vi "Create Server.vi"(5 "Server Key File (.key)":path, 7 "Server Certificate File (.crt)":path, 8 "error in (no error)":errorcluster, 11 "Server Address":string) -> (0 "error out":errorcluster, 3 "gRPC Server out":refnum<class "HVC4.lvclass">)   [LabVIEW 2019, in "HVC4.lvlib" / "HVC4.lvclass"]
uses:
  HVC4.lvclass
  HVC4.lvclass/HVC4.ctl
  gRPC lvSupport/gprc-lvsupport.lvlib
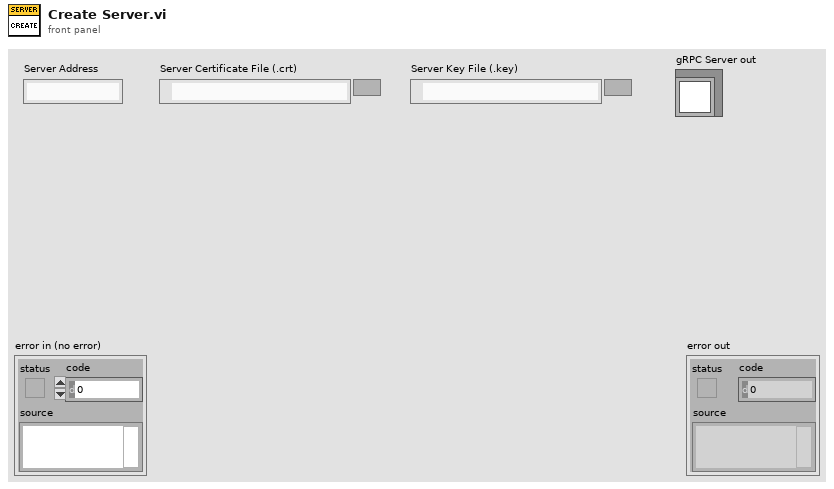
[diagram p1: front panel]
types:
  T1 = typedef "HVC4.lvlib/gprc-lvsupport.lvlib/grpcId.ctl" = u64
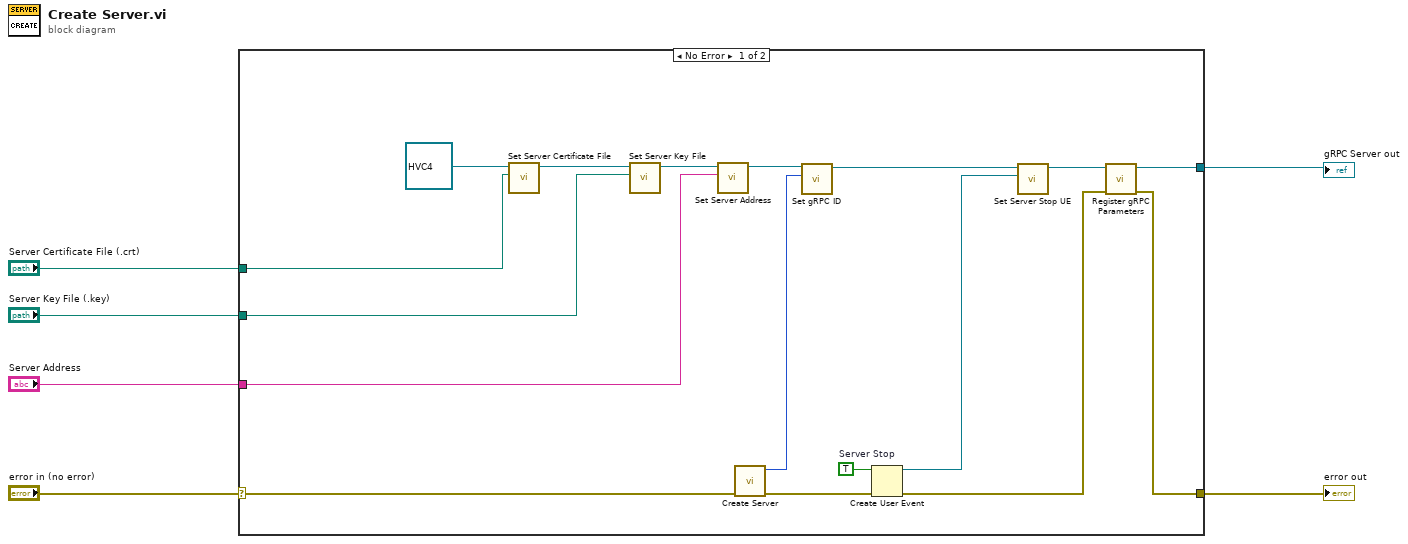
[diagram p0: block diagram]
diagram:
  n1 = case shown="No Error" "error in (no error)" {
    selector: "error in (no error)" -> [w23 w24]
    tunnel: [w7 w24] -> w5
    tunnel: [w9 _] -> w4
    tunnel: "Server Certificate File (.crt)" -> [w18 _]
    tunnel: "Server Key File (.key)" -> [w17 _]
    tunnel: "Server Address" -> [w16 _]
    frame No Error {
      w14 = TRUE  # Server Stop
      n2 = call "Set Server Certificate File.vi"("Server Certificate File (.crt)"=w18, "OOP Server in"=refnum<class "HVC4.lvclass"> refnum ("OOP Server out")) -> ("OOP Server out"=w21:refnum<class "HVC4.lvclass">)  [unwired: 9 in]
      n3 = call "Set Server Key File.vi"("Server Key File (.key)"=w17, "OOP Server in"=w21) -> ("OOP Server out"=w20:refnum<class "HVC4.lvclass">)  [unwired: 9 in]
      n4 = call "Set Server Address.vi"("Server Address"=w16, "OOP Server in"=w20) -> ("OOP Server out"=w19:refnum<class "HVC4.lvclass">)  [unwired: 9 in]
      n5 = call "Create Server.vi"("error in (no error)"=w23) -> ("error out"=w12:errorcluster, "gRPCid"=w15:T1)  [unwired: 9 in]
      n6 = call "Set gRPC ID.vi"("gRPC ID"=w15, "OOP Server in"=w19) -> ("OOP Server out"=w13:refnum<class "HVC4.lvclass">)  [unwired: 9 in]
      n7 = Create User Event(user event datatype=w14, error in=w12) -> (user event=w11:refnum<user-event>, error out=w8:errorcluster)
      n8 = call "Set Server Stop UE.vi"("Server Stop UE"=w11, "OOP Server in"=w13) -> ("OOP Server out"=w10:refnum<class "HVC4.lvclass">)  [unwired: 9 in]
      n9 = call "Register gRPC Parameters.vi"("error in (no error)"=w8, "OOP Server in"=w10) -> ("error out"=w7:errorcluster, "OOP Server out"=w9:refnum<class "HVC4.lvclass">)  [unwired: 8 in]
    }
    frame Error {
    }
  }
  "error out" <- w5
  "gRPC Server out" <- w4
